vi "Accelerator DML GEMM And Operations.vi"(9 "Sessions Parameters":T2={"intra_op_num_threads"=0, "inter_op_num_threads"=0, "execution_mode"=enum."ORT_SEQUENTIAL", "deterministic_compute"=FALSE, "graph_optimization_level"=1, "optimized_model_file_path"=path "", "profiling output dir"=path ""} {"graph_optimization_level" items=["ORT_DISABLE_ALL"=0, "ORT_ENABLE_ALL"=1, "ORT_ENABLE_BASIC"=2, "ORT_ENABLE_EXTENDED"=99]}, 11 "dimension size":i32=16384) -> (3 "Accelerator Time":dbl=0.19947869999998602)   [LabVIEW 2020]
uses:
  <vilib>/Graiphic/Accelerator/Source/Layer/Node/Gemm/_Controls/acc_gemm_param.ctl
  <vilib>/Graiphic/Accelerator/Source/Model/Controls/acc_input_parameters.ctl
  <vilib>/Graiphic/Accelerator/Source/Layer/Node/_Controls/acc_onnx_dtype_enum.ctl
  <vilib>/Graiphic/Accelerator/Source/SubVIs/add_to_cluster_onnx_input/acc_onnx_add_2d_float_array_into_input_cluster_array_by_idx.vi
  <vilib>/Graiphic/Accelerator/Source/Model/_Methods/add_to_graph/Initializer/acc_float_scalar_initializer.vi
  <vilib>/Graiphic/Accelerator/Source/Model/_Methods/add_to_graph/Numeric/acc_add_adaptive.vi
  <vilib>/Graiphic/Accelerator/Source/Model/_Methods/acc_create_onnx_model_then_init_dml_inference_session.vi
  <vilib>/Graiphic/Accelerator/Source/SubVIs/add_to_cluster_onnx_input/acc_onnx_add_scalar_float_into_input_cluster_array_by_idx.vi
  <vilib>/Graiphic/Accelerator/Source/ONNX/Inference/_Methods/Simplified/acc_embedded_run_preallocated_multi_input_and_outputs_dml_by_idx.vi
  <vilib>/Graiphic/Accelerator/Source/ONNX/Inference/_Methods/Exec_DML/acc_embedded_copy_dml_ptr_data_to_labview_data.vi
  <vilib>/Graiphic/Accelerator/Source/ONNX/Inference/_Methods/Simplified/acc_embedded_run_mono_output_scalar_float.vi
  <vilib>/Graiphic/Accelerator/Source/ONNX/Inference/acc_Inference.lvclass
  <vilib>/Graiphic/Accelerator/Source/Model/acc_Model.lvclass
  <vilib>/Analysis/NI_AALBase.lvlib
panel:
  in  "Parameters":T1={"alpha"=1.0, "beta"=0.0, "transA"=0, "transB"=0}
  out "max value":sgl=5.4420166
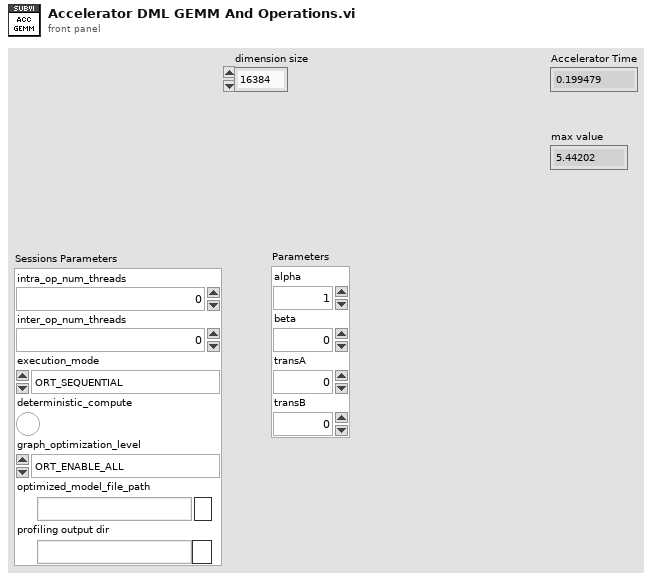
[diagram p1: front panel]
types:
  T1 = typedef "acc_gemm_param.ctl" = cluster{"alpha":sgl, "beta":sgl, "transA":i64, "transB":i64}
  T2 = cluster{"intra_op_num_threads":i32, "inter_op_num_threads":i32, "execution_mode":enum16{"ORT_SEQUENTIAL", "ORT_PARALLEL"}, "deterministic_compute":bool, "graph_optimization_level":u16, "optimized_model_file_path":path, "profiling output dir":path}
  T3 = typedef "acc_input_parameters.ctl" = cluster{"Rank":enum16{"Scalar", "1D", "2D", "3D", "4D", "5D", "6D"}, "dtype":T4, "complex?":bool, "expert?":bool}
  T4 = typedef "acc_onnx_dtype_enum.ctl" = enum16{"UNDEFINED", "FLOAT", "UINT8", "INT8", "UINT16", "INT16", "INT32", "INT64", "STRING", "BOOL", "FLOAT16", "DOUBLE", "UINT32", "UINT64", "COMPLEX64", "COMPLEX128", "BFLOAT16", "FLOAT8E4M3FN", "FLOAT8E4M3FNUZ", "FLOAT8E5M2", "FLOAT8E5M2FNUZ", "UINT4", "INT4"}
  T5 = typedef "acc_onnx_multi_input_index_cluster.ctl" = cluster{"input_order":u32, "Inputs Info":cluster{"inputs_data":u8[], "inputs_shapes":i64[], "inputs string length":i64[], "inputs_ranks":i64[], "inputs_types":T4[]}}
  T6 = typedef "acc_onnx_multi_ptr_input_index_cluster.ctl" = cluster{"input_order":u32, "Inputs Info":cluster{"inputs_ptr":u64, "inputs_shapes":i64[], "inputs_ranks":i64, "inputs_types":T4}}
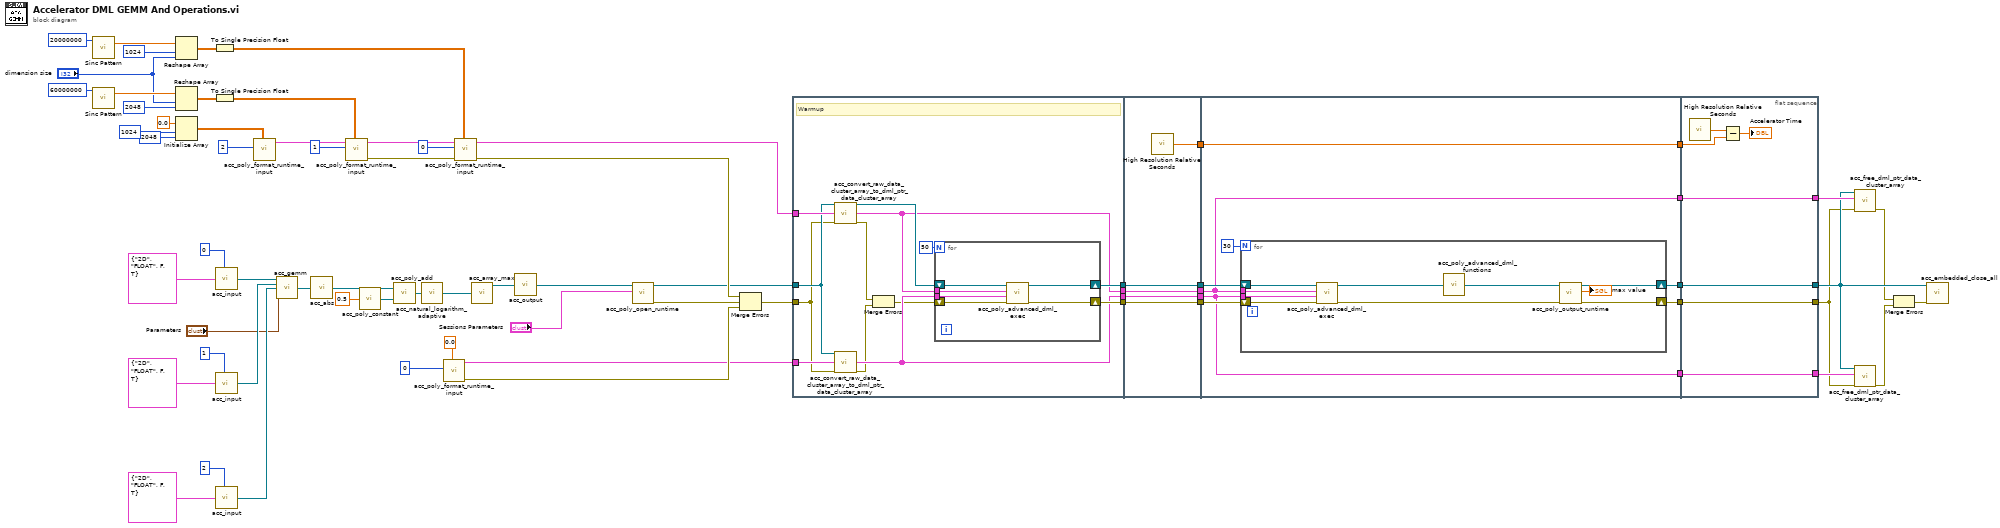
[diagram p0: block diagram]
diagram:
  n1 = call <vilib>:"Sinc Pattern.vi"("samples"=20000000) -> ("Sinc Pattern"=w52:dbl[])  [unwired: 3 in, 1 out]
  n2 = call <vilib>:"Sinc Pattern.vi"("samples"=60000000) -> ("Sinc Pattern"=w51:dbl[])  [unwired: 3 in, 1 out]
  n3 = Reshape Array(w52, 1024 ("dimension size"), "dimension size") -> (w47:dbl[][])
  n4 = Reshape Array(w51, "dimension size", 2048 ("dimension size")) -> (w46:dbl[][])
  n5 = Initialize Array(sgl 0.0 ("element"), 1024 ("dimension size"), 2048 ("dimension size")) -> (w17:sgl[][])
  n6 = To Single Precision Float(number=w47) -> (single precision float=w18:sgl[][])
  n7 = To Single Precision Float(number=w46) -> (single precision float=w16:sgl[][])
  n8 = call <vilib>:"acc_input.vi"("index"=0, "Parameters"=T3 {"Rank"=enum."2D", "dtype"=enum."FLOAT", "complex?"=FALSE, "expert?"=TRUE}) -> ("ONNXModel out"=w34:refnum<class "acc_Model.lvclass">)  [unwired: 7 in]
  n9 = call <vilib>:"acc_input.vi"("index"=1, "Parameters"=T3 {"Rank"=enum."2D", "dtype"=enum."FLOAT", "complex?"=FALSE, "expert?"=TRUE}) -> ("ONNXModel out"=w33:refnum<class "acc_Model.lvclass">)  [unwired: 7 in]
  n10 = call <vilib>:"acc_input.vi"("index"=2, "Parameters"=T3 {"Rank"=enum."2D", "dtype"=enum."FLOAT", "complex?"=FALSE, "expert?"=TRUE}) -> ("ONNXModel out"=w25:refnum<class "acc_Model.lvclass">)  [unwired: 7 in]
  n11 = call-poly <vilib>:"acc_poly_format_runtime_input.vi"("2D Input Data"=w17, "input order"=2) -> ("Data out (Fwd in)"=w23:T5[])  [unwired: 8 in, 1 out]
  n12 = call <vilib>:"acc_gemm.vi"("A"=w34, "B"=w33, "C"=w25, "Parameters"="Parameters") -> ("subarray"=w32:refnum<class "acc_Model.lvclass">)  [unwired: 11 in]
  n13 = call <vilib>:"acc_abs.vi"("x"=w32) -> ("abs(x)"=w22:refnum<class "acc_Model.lvclass">)
  n14 = call-poly <vilib>:"acc_poly_format_runtime_input.vi"("2D Input Data"=w16, "input order"=1, "Data in"=w23) -> ("error out"=w40:errorcluster, "Data out (Fwd in)"=w41:T5[])  [unwired: 7 in]
  n15 = call-poly <vilib>:"acc_poly_constant.vi"("scalar"=sgl 0.5) -> ("Float Scalar"=w20:refnum<class "acc_Model.lvclass">)  [unwired: 3 in]
  n16 = call-poly <vilib>:"acc_poly_add.vi"("y"=w20, "x"=w22) -> ("x+y"=w19:refnum<class "acc_Model.lvclass">)
  n17 = call <vilib>:"acc_natural_logarithm_adaptive.vi"("x"=w19) -> ("ln(x)"=w35:refnum<class "acc_Model.lvclass">)
  n18 = call-poly <vilib>:"acc_poly_format_runtime_input.vi"("Input Data"=sgl 0.0, "input order"=0) -> ("error out"=w38:errorcluster, "Data out (Fwd in)"=w15:T5[])  [unwired: 8 in]
  n19 = call-poly <vilib>:"acc_poly_format_runtime_input.vi"("2D Input Data"=w18, "error in"=w40, "input order"=0, "Data in"=w41) -> ("error out"=w39:errorcluster, "Data out (Fwd in)"=w14:T5[])  [unwired: 6 in]
  n20 = call <vilib>:"acc_array_max.vi"("array"=w35) -> ("max value"=w48:refnum<class "acc_Model.lvclass">)  [unwired: 6 in, 1 out]
  n21 = call <vilib>:"acc_output.vi"("ONNXModel in"=w48) -> ("ONNXModel out"=w8:refnum<class "acc_Model.lvclass">)  [unwired: 8 in]
  n22 = call-poly <vilib>:"acc_poly_open_runtime.vi"("Sessions Parameters"="Sessions Parameters", "Model in"=w8) -> ("error out"=w10:errorcluster, "Inference out"=w11:refnum<class "acc_Inference.lvclass">)  [unwired: 8 in]
  n23 = Merge Errors(w39, w10, w38) -> (w37:errorcluster)
  n24 = flat-sequence {
    tunnel: w37 -> [w74]
    tunnel: w14 -> [w79]
    tunnel: w15 -> [w78]
    tunnel: w11 -> [w77]
    tunnel: [w83] -> w70
    tunnel: [w76] -> w69
    tunnel: [w82] -> w68
    tunnel: [w75] -> w67
    tunnel: [w94] -> w66
    tunnel: [w93] -> w65
    tunnel: [w92] -> w64
    tunnel: [w91] -> w63
    tunnel: [w90] -> w62
    tunnel: w70 -> [w93]
    tunnel: w69 -> [w92]
    tunnel: w68 -> [w90]
    tunnel: w67 -> [w91]
    tunnel: w66 -> [w102]
    tunnel: [w102] -> w61
    tunnel: w65 -> [w100]
    tunnel: w64 -> [w95]
    tunnel: w63 -> [w96]
    tunnel: w62 -> [w99]
    tunnel: [w98] -> w60
    tunnel: [w97] -> w59
    tunnel: [w96] -> w58
    tunnel: [w95] -> w57
    tunnel: w61 -> [w118]
    tunnel: [w116] -> w5
    tunnel: w60 -> [w116]
    tunnel: w59 -> [w115]
    tunnel: [w115] -> w1
    tunnel: [w114] -> w13
    tunnel: w58 -> [w114]
    tunnel: [w113] -> w12
    tunnel: w57 -> [w113]
    frame #0 {
      # "Warmup"
      n25 = call <vilib>:"acc_convert_raw_data_cluster_array_to_dml_ptr_data_cluster_array.vi"("Inference in"=w77, "Data in"=w79, "error in"=w74) -> ("Inference out"=w80:refnum<class "acc_Inference.lvclass">, "Data in"=w75:T6[], "error out"=w71:errorcluster)  [unwired: 10 in]
      n26 = call <vilib>:"acc_convert_raw_data_cluster_array_to_dml_ptr_data_cluster_array.vi"("Inference in"=w77, "Data in"=w78, "error in"=w74) -> ("Data in"=w76:T6[], "error out"=w73:errorcluster)  [unwired: 10 in, 1 out]
      n27 = Merge Errors(w71, w73) -> (w72:errorcluster)
      n28 = for {
        N: 50 -> [_]
        tunnel: w75 -> [w86]
        tunnel: w76 -> [w85]
        shift-right: [w88] -> w83
        shift-left: w80 -> [w89]
        shift-right: [w84] -> w82
        shift-left: w72 -> [w87]
        n29 = call-poly <vilib>:"acc_poly_advanced_dml_exec.vi"("error in"=w87, "Data out"=w85, "Data in"=w86, "Inference in"=w89) -> ("error out"=w84:errorcluster, "Inference out"=w88:refnum<class "acc_Inference.lvclass">)  [unwired: 6 in]
      }
    }
    frame #1 {
      n30 = call <vilib>:"High Resolution Relative Seconds.vi"() -> ("relative seconds"=w94:dbl)
    }
    frame #2 {
      n31 = for {
        N: 30 -> [_]
        tunnel: w95 -> [w111]
        tunnel: w96 -> [w110]
        shift-right: [w106] -> w98
        shift-left: w100 -> [w112]
        shift-right: [w105] -> w97
        shift-left: w99 -> [w109]
        n32 = call-poly <vilib>:"acc_poly_advanced_dml_exec.vi"("error in"=w109, "Data out"=w111, "Data in"=w110, "Inference in"=w112) -> ("error out"=w107:errorcluster, "Inference out"=w108:refnum<class "acc_Inference.lvclass">)  [unwired: 6 in]
        n33 = call-poly <vilib>:"acc_poly_advanced_dml_functions.vi"("Inference in"=w108) -> ("Inference out"=w104:refnum<class "acc_Inference.lvclass">)
        n34 = call-poly <vilib>:"acc_poly_output_runtime.vi"("error in"=w107, "Inference in"=w104) -> ("error out"=w105:errorcluster, "Output Data"=→"max value":sgl, "Inference out"=w106:refnum<class "acc_Inference.lvclass">)  [unwired: 7 in]
      }
    }
    frame #3 {
      n35 = call <vilib>:"High Resolution Relative Seconds.vi"() -> ("relative seconds"=w119:dbl)
      n36 = Subtract(x=w119, y=w118) -> (x-y=→"Accelerator Time":dbl)
    }
  }
  n37 = call <vilib>:"acc_free_dml_ptr_data_cluster_array.vi"("error in"=w1, "Data in"=w13, "Inference in"=w5) -> ("error out"=w3:errorcluster)  [unwired: 7 in, 1 out]
  n38 = call <vilib>:"acc_free_dml_ptr_data_cluster_array.vi"("error in"=w1, "Data in"=w12, "Inference in"=w5) -> ("error out"=w4:errorcluster)  [unwired: 7 in, 1 out]
  n39 = Merge Errors(w3, w4) -> (w2:errorcluster)
  n40 = call-dynamic "acc_embedded_close_all.vi"("error in"=w2, "Inference in"=w5) -> ()  [unwired: 8 in, 2 out]
